vi "Array_Coords_to_Index.vi"(6 "coords":cluster{"Horizontal":i32, "Vertical":i32}, 7 "Array ref":refnum<vi>) -> (0 "H In Range?":bool, 1 "col index":i16, 2 "V In Range?":bool, 3 "row index":i16)   [LabVIEW 2020]
doc: "Given a reference to a 1-D or 2-D array, and screen coordinates,\nreturn the index of the element at that location.\nTwo values are returned: col index is valid for horizontal arrays, and row index is valid for vertical arrays, both are valid for 2-D arrays"
panel:
  in  "error in (no error)":errorcluster
  out "error out":errorcluster
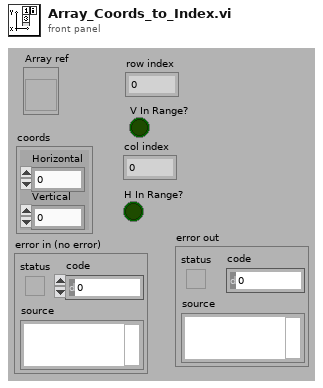
[diagram p1: front panel]
types:
  T1 = typedef "LVRectTypeDef.ctl" = cluster{"Left":i16, "Top":i16, "Right":i16, "Bottom":i16}
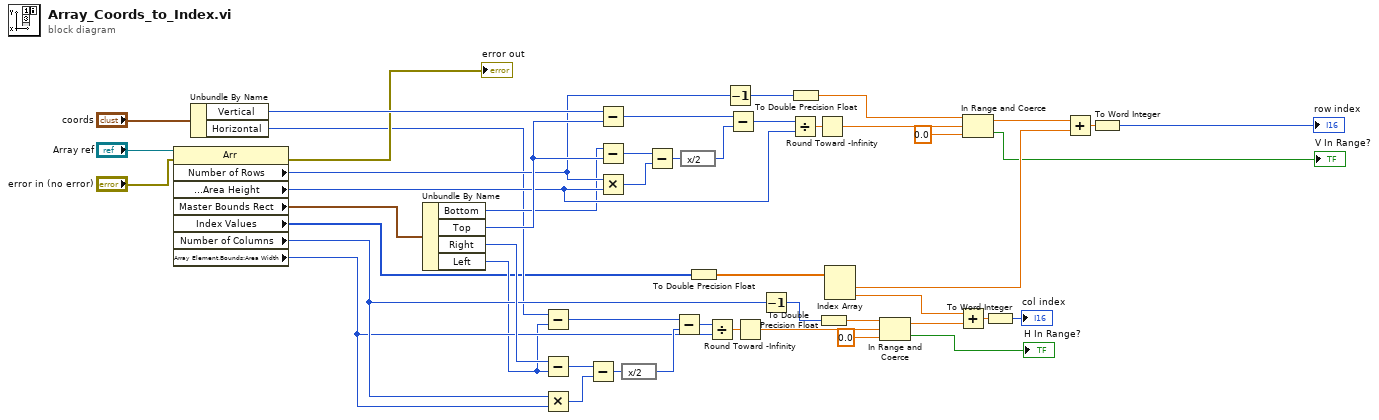
[diagram p0: block diagram]
diagram:
  n1 = property on="Property Node" class="Arr"(reference="Array ref", error in="error in (no error)") -> (error out=→"error out":errorcluster, "Number of Rows"=w11:u32, "Array Element.Bounds:Area Height"=w18:u32, "Master Bounds Rect"=w10:T1, "Index Values"=w6:u32[], "Number of Columns"=w14:u32, "Array Element.Bounds:Area Width"=w13:u32)  [unwired: 1 out]
  n2 = Unbundle By Name("coords") -> ("Vertical"=w44:i32, "Horizontal"=w7:i32)
  n3 = Unbundle By Name(w10) -> ("Bottom"=w9:i16, "Top"=w20:i16, "Right"=w15:i16, "Left"=w8:i16)
  n4 = Subtract(x=w7, y=w8) -> (x-y=w30:i32)
  n5 = Subtract(x=w15, y=w8) -> (x-y=w17:i16)
  n6 = Multiply(x=w14, y=w13) -> (x*y=w33:u32)
  n7 = Subtract(x=w17, y=w33) -> (x-y=w32:u32)
  n8 = Subtract(x=w44, y=w20) -> (x-y=w25:i32)
  n9 = Subtract(x=w9, y=w20) -> (x-y=w19:i16)
  n10 = Multiply(x=w11, y=w18) -> (x*y=w27:u32)
  n11 = expression code="x/2"(w32) -> (w31:u32)
  n12 = Subtract(x=w19, y=w27) -> (x-y=w28:u32)
  n13 = Subtract(x=w30, y=w31) -> (x-y=w29:u32)
  n14 = expression code="x/2"(w28) -> (w26:u32)
  n15 = To Double Precision Float(number=w6) -> (double precision float=w2:dbl[])
  n16 = Divide(x=w29, y=w13) -> (x/y=w36:dbl)
  n17 = Decrement(x=w11) -> (x-1=w46:u32)
  n18 = Subtract(x=w25, y=w26) -> (x-y=w24:u32)
  n19 = Round Toward -Infinity(1:w36) -> (0:w22:dbl)
  n20 = Decrement(x=w14) -> (x-1=w41:u32)
  n21 = Divide(x=w24, y=w18) -> (x/y=w37:dbl)
  n22 = To Double Precision Float(number=w46) -> (double precision float=w1:dbl)
  n23 = Round Toward -Infinity(1:w37) -> (0:w23:dbl)
  n24 = To Double Precision Float(number=w41) -> (double precision float=w3:dbl)
  n25 = Index Array(array=w2) -> (element #1=w48:dbl, element #2=w4:dbl)  [unwired: 2 in]
  n26 = In Range and Coerce(upper limit=w3, x=w22, lower limit=0.0) -> (coerced(x)=w5:dbl, In Range?=→"H In Range?":bool)
  n27 = Add(x=w4, y=w5) -> (x+y=w42:dbl)
  n28 = In Range and Coerce(upper limit=w1, x=w23, lower limit=0.0) -> (coerced(x)=w49:dbl, In Range?=→"V In Range?":bool)
  n29 = To Word Integer(number=w42) -> (16bit integer=→"col index":i16)
  n30 = Add(x=w49, y=w48) -> (x+y=w47:dbl)
  n31 = To Word Integer(number=w47) -> (16bit integer=→"row index":i16)
